vi "Arduino to LabVIEW Communication Modue Complex.vi"() -> ()   [LabVIEW 2018]
uses:
  TypeDeclarations/GEVE Ventilator Monitoring Data.ctl
  <vilib>/Instr/_visa.llb/VISA Configure Serial Port (Instr).vi
  TypeDeclarations/Serial Port Configuration.ctl
panel:
  out "GEVE Ventilator Monitoring Data":T1
  out "loop time (ms)":u32
  out "Waveform Chart":u32(graph)
  out "read buffer data byte array":u8[](array[numeric]) format="%02x"
  in  "baud rate (9600)":u32=9600
  out "Communication Timeout?":bool
  in  "VISA resource name":refnum<visa-resource-name>="COM7"
  out "return count read":u32
  out "read buffer":string
  in  "Stop":bool
  out "Iterations":i32
  # "DEBUG AREA"
  # "iterations"
  # "poti"
  # "pressure"
  # "alarm"
  # "EOL"
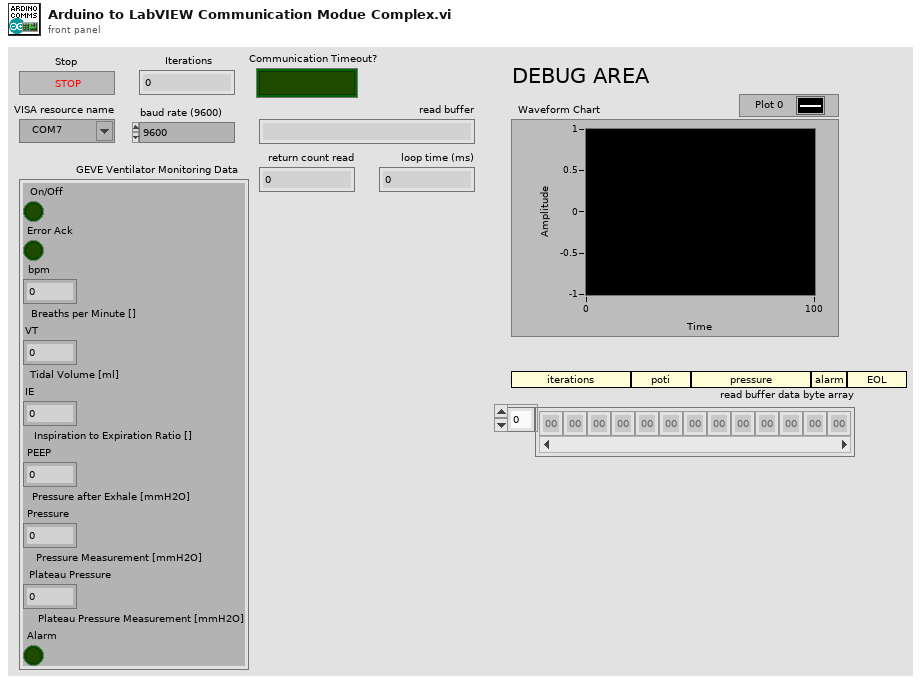
[diagram p1: front panel]
types:
  T1 = typedef "GEVE Ventilator Monitoring Data.ctl" = cluster{"On/Off":bool, "Error Ack":bool, "bpm":dbl, "VT":dbl, "IE":dbl, "PEEP":dbl, "Pressure":dbl, "Plateau Pressure":dbl, "Alarm":bool}
  T2 = typedef "Serial Port Configuration.ctl" = cluster{"timeout (ms)":u32, "VISA resource name":refnum<visa-resource-name>, "baud rate":u32}
  T3 = cluster{"GEVE Ventilator Monitoring Data":T1, "Serial Port Configuration":T2, "Application Events":cluster{"Serial Port Config event":refnum<user-event>}}
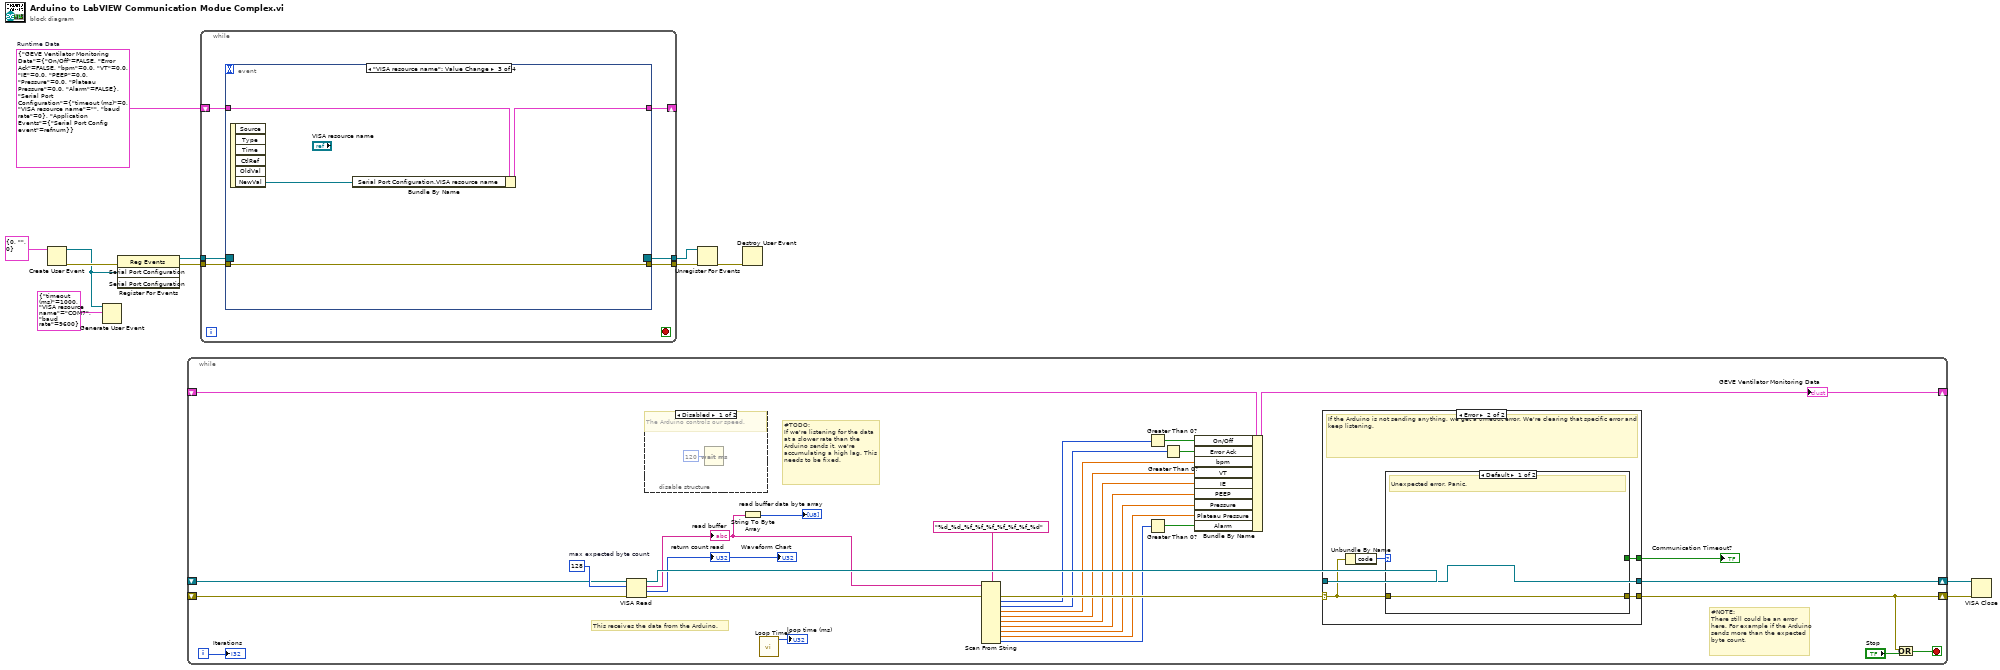
[diagram p0: block diagram]
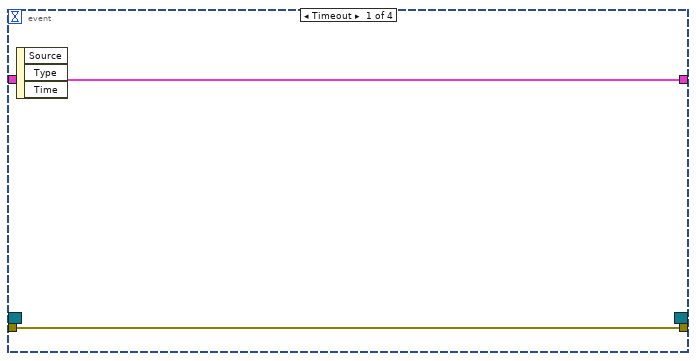
[diagram p2: hidden frame]
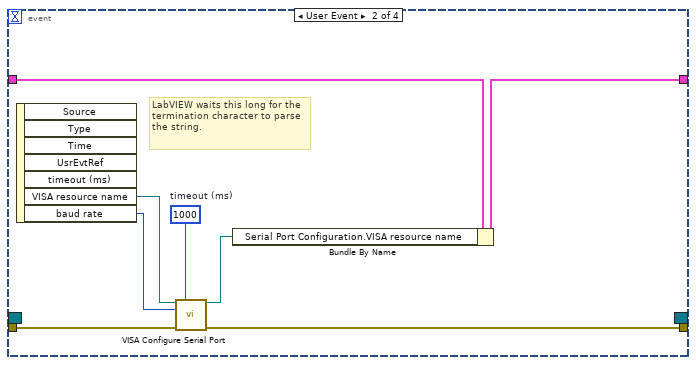
[diagram p3: hidden frame]
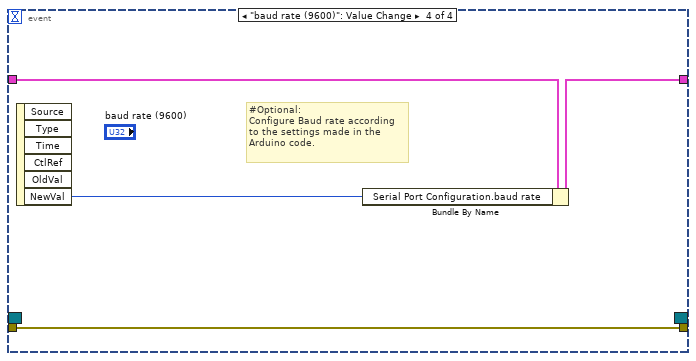
[diagram p4: hidden frame]
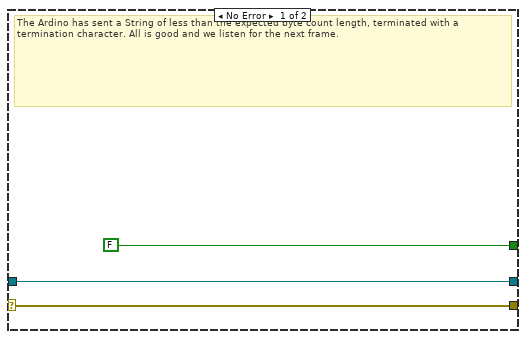
[diagram p6: hidden frame]
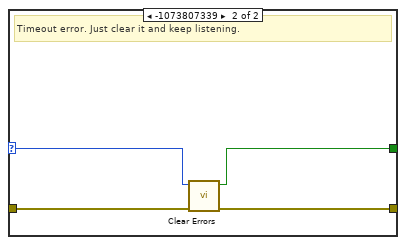
[diagram p7: hidden frame]
diagram:
  w1 = T3 {"GEVE Ventilator Monitoring Data"={"On/Off"=FALSE, "Error Ack"=FALSE, "bpm"=0.0, "VT"=0.0, "IE"=0.0, "PEEP"=0.0, "Pressure"=0.0, "Plateau Pressure"=0.0, "Alarm"=FALSE}, "Serial Port Configuration"={"timeout (ms)"=0, "VISA resource name"="", "baud rate"=0}, "Application Events"={"Serial Port Config event"=refnum}}  # Runtime Data
  n1 = Create User Event(user event datatype=T2 {"timeout (ms)"=0, "VISA resource name"="", "baud rate"=0} ("Serial Port Configuration")) -> (user event=w3:refnum<user-event>, error out=w5:errorcluster)  [unwired: 1 in]
  n2 = Generate User Event(user event=w3, event data cluster=T2 {"timeout (ms)"=1000, "VISA resource name"="COM7", "baud rate"=9600} ("event data")) -> ()  [unwired: 2 in, 2 out]
  n3 = register-events(error in=w5, w3) -> (reference out=w9:refnum<event-registration>, error out=w10:errorcluster)  [unwired: 2 in]
  n4 = while {
    shift-right: [w38] -> w12
    shift-left: _ -> [w30]
    shift-right: [w39] -> w11
    shift-left: _ -> [w29]
    shift-right: [w25] -> _
    shift-left: _ -> [w26]
    i -> [w43]
    stop <- w41 stop-if-true
    w40 = u32 128  # max expected byte count
    # "#TODO:\nIf we're listening for the data at a slower rate than the Arduino sends it, we're accumulating a high lag. This needs to be fixed."
    # "This receives the data from the Arduino."
    # "#NOTE:\nThere still could be an error here. For example if the Arduino sends more than the expected byte count."
    n5 = VISA Read(VISA resource name=w30, byte count=w40, error in (no error)=w29) -> (VISA resource name out=w37:refnum<visa-resource-name>, read buffer=w32:string, return count=→"return count read" →"Waveform Chart":u32, error out=w31:errorcluster)
    "read buffer" <- w32
    n6 = disable-structure shown="Disabled" {
      frame Disabled {
        # "The Arduino controls our speed."
        n7 = Wait (ms)(milliseconds to wait=u32 120) -> ()  [unwired: 1 out]
      }
      frame Enabled {
      }
    }
    n8 = String To Byte Array(string=w32) -> (unsigned byte array=→"read buffer data byte array":u8[])
    n9 = call "Loop Timer.vi"() -> ("loop time (ms)"=→"loop time (ms)":u32)  [unwired: 11 in]
    n10 = Scan From String(format string="%d_%d_%f_%f_%f_%f_%f_%f_%d", input string=w32, error in=w31) -> (error out=w35:errorcluster, output 1=w23:i32, output 2=w22:i32, output 3=w27:dbl, output 4=w14:dbl, output 5=w15:dbl, output 6=w16:dbl, output 7=w17:dbl, output 8=w18:dbl, output 9=w24:i32)  [unwired: 10 in, 2 out]
    n11 = Greater Than 0?(x=w23) -> (x > 0?=w21:bool)
    n12 = Greater Than 0?(x=w24) -> (x > 0?=w19:bool)
    n13 = Greater Than 0?(x=w22) -> (x > 0?=w20:bool)
    n14 = Bundle By Name(cluster=w26, "On/Off"=w21, "Error Ack"=w20, "bpm"=w27, "VT"=w14, "IE"=w15, "PEEP"=w16, "Pressure"=w17, "Plateau Pressure"=w18, "Alarm"=w19) -> (w25:cluster{})
    "GEVE Ventilator Monitoring Data" <- w25
    n15 = case shown="Error" w35 {
      selector: w35 -> [w47 w49]
      tunnel: [w47 w52] -> w39
      tunnel: [w46 w51] -> w38
      tunnel: w37 -> [w46 w51]
      tunnel: [FALSE ("specific error cleared?") w50] -> w36
      frame No Error {
        # "The Ardino has sent a String of less than the expected byte count length, terminated with a termination character. All is good and we listen for the next frame."
      }
      frame Error {
        # "If the Arduino is not sending anything, we get a timeout error. We're clearing that specific error and keep listening."
        n16 = Unbundle By Name(w49) -> ("code"=w48:i32)
        n17 = case shown="Default" w48 {
          selector: w48 -> [_ w55]
          tunnel: w49 -> [w53 w57]
          tunnel: [w53 w56] -> w52
          tunnel: [_ w54] -> w50
          frame Default {
            # "Unexpected error. Panic."
          }
          frame -1073807339 {
            # "Timeout error. Just clear it and keep listening."
            n18 = call <vilib>:"Clear Errors.vi"("error in (no error)"=w57, "specific error code to clear (0: all)"=w55) -> ("error out"=w56:errorcluster, "specific error cleared?"=w54:bool)  [unwired: 4 in]
          }
        }
      }
    }
    "Communication Timeout?" <- w36
    n19 = Or(x=w39, y="Stop") -> (x .or. y?=w41:bool)
    "Iterations" <- w43
  }
  n20 = while {
    shift-right: [w63] -> _
    shift-left: w1 -> [w62]
    tunnel: [w61] -> w7
    tunnel: w10 -> [w60]
    tunnel: w9 -> [w59]
    tunnel: [w58] -> w8
    stop <- _ stop-if-true
    n21 = event shown="[2] \"VISA resource name\": Value Change" {
      selector: w59 -> [_ _ _ _]
      dyn-events: [_ _ _ _] -> w58
      timeout: _ -> [_ _ _ _]
      tunnel: [w65 w66 w74 w79] -> w63
      tunnel: w62 -> [w65 w68 w76 w80]
      tunnel: [w64 w70 w77 w81] -> w61
      tunnel: w60 -> [w64 w71 w77 w81]
      event Timeout {
        n22 = event-data() -> ()  [unwired: 1 in, 3 out]
      }
      event User Event {
        w69 = u32 1000  # timeout (ms)
        # "LabVIEW waits this long for the termination character to parse the string."
        n23 = event-data() -> ("VISA resource name"=w73:refnum<visa-resource-name>, "baud rate"=w72:u32)  [unwired: 1 in, 5 out]
        n24 = call-poly "VISA Configure Serial Port"("VISA resource name"=w73, "timeout (10sec)"=w69, "baud rate (9600)"=w72, "error in (no error)"=w71) -> ("VISA resource name out"=w67:refnum<visa-resource-name>, "error out"=w70:errorcluster)  [unwired: 10 in]
        n25 = Bundle By Name(cluster=w68, "Serial Port Configuration.VISA resource name"=w67) -> (w66:T3)
      }
      event "VISA resource name": Value Change {
        n26 = event-data() -> ("NewVal"=w75:refnum<visa-resource-name>)  [unwired: 1 in, 5 out]
        n27 = Bundle By Name(cluster=w76, "Serial Port Configuration.VISA resource name"=w75) -> (w74:T3)
      }
      event "baud rate (9600)": Value Change {
        # "#Optional:\nConfigure Baud rate according to the settings made in the Arduino code."
        n28 = event-data() -> ("NewVal"=w78:u32)  [unwired: 1 in, 5 out]
        n29 = Bundle By Name(cluster=w80, "Serial Port Configuration.baud rate"=w78) -> (w79:T3)
      }
    }
  }
  n30 = Unregister For Events(event registration refnum=w8, error in=w7) -> (error out=w6:errorcluster)
  n31 = Destroy User Event(error in=w6) -> ()  [unwired: 1 in, 1 out]
  n32 = VISA Close(VISA resource name=w12, error in (no error)=w11) -> ()  [unwired: 1 out]
